vi "Record location.vi"() -> ()   [LabVIEW 2016]
uses:
  Classes/Controllers/Camera/Copy of Camera Folder/Machine Vision.ctl
  Classes/Controllers/Motion/Copy of A3200 Folder/A3200.lvclass
  <vilib>/Utility/file.llb/Read Delimited Spreadsheet (DBL).vi
  <vilib>/Utility/file.llb/Write Delimited Spreadsheet (DBL).vi
  Classes/Controllers/Motion/Copy of Motion Folder/Motion.lvclass
  Classes/Controllers/Camera/Copy of Camera Folder/Camera.lvclass
  Classes/Controllers/Camera/Copy of Controller Folder/Controller.lvclass
panel:
  out "Sum 2":dbl[](array[numeric])
  out "Gantry 2":dbl[](array[numeric])
  out "Camera 2":dbl[](array[numeric])
  in  "Record":bool
  out "XYZTheta Out":dbl[](array[numeric])
  in  "stop":bool
  in  "start":bool
  in  "Speed 1":dbl
  out "XYZTheta Out 2":dbl[](array[numeric])
  in  "file path":path
  out "first row":dbl[](array[numeric])
  out "all rows":dbl[][](array[numeric])
  in  "Z Go":bool
  in  "Position":dbl
  in  "Go":bool
  in  "XYZTheta":dbl[](array[numeric])
  in  "Joystick":bool
  out "Gantry":dbl[](array[numeric])
  out "Sum":dbl[](array[numeric])
  in  "Stop":bool
  out "Image":T1(plugin-control)
  out "Camera":dbl[](array[numeric])
  in  "Machine Vision":T2=enum."None"
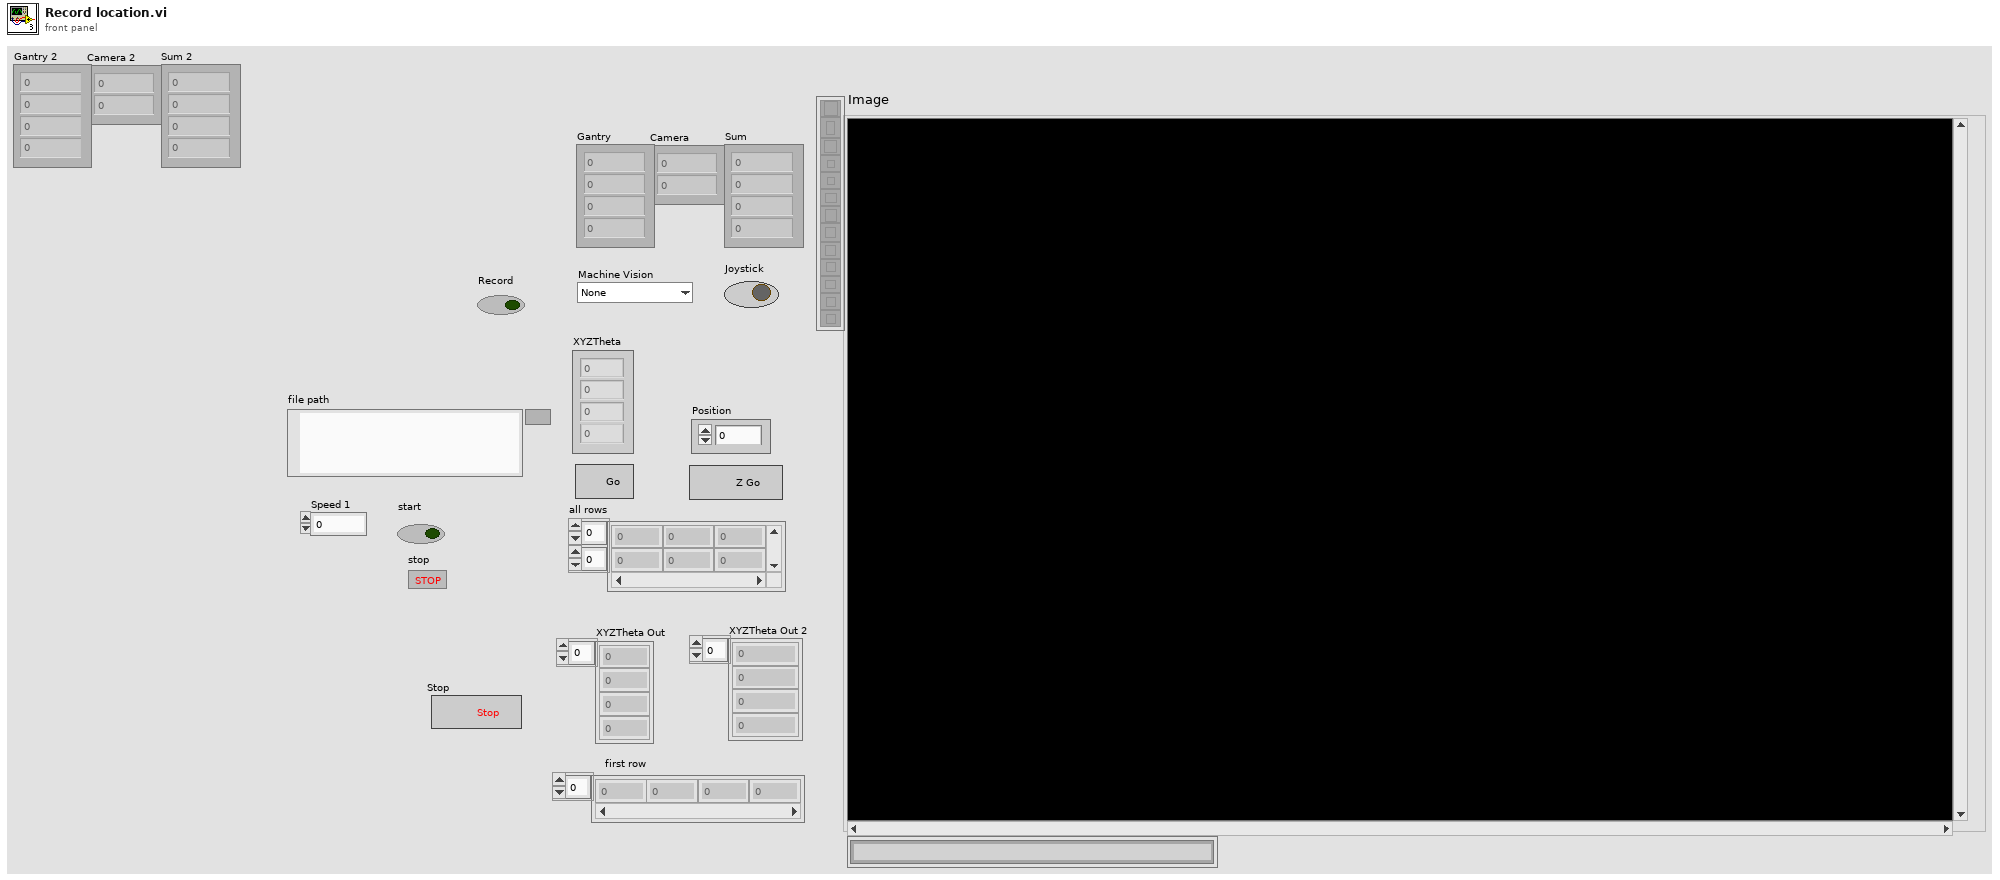
[diagram p1: front panel]
types:
  T1 = typedef "IMAQ Image.ctl" = refnum<image>
  T2 = typedef "Camera.lvclass/Machine Vision.ctl" = enum16{"Focus", "LargeCircle", "None", "INTT HDI Mark", "INTT Sensor Cross", "INTT Chip Corner", "HPK Silicon", "circle"}
  T3 = typedef "Controller.lvclass/Controllers.ctl" = cluster{"Copy of Motion.lvclass":refnum<class "Motion.lvclass">, "Copy of I-O.lvclass":refnum<class "I-O.lvclass">, "Copy of Dispenser.lvclass":refnum<class "Dispenser.lvclass">}
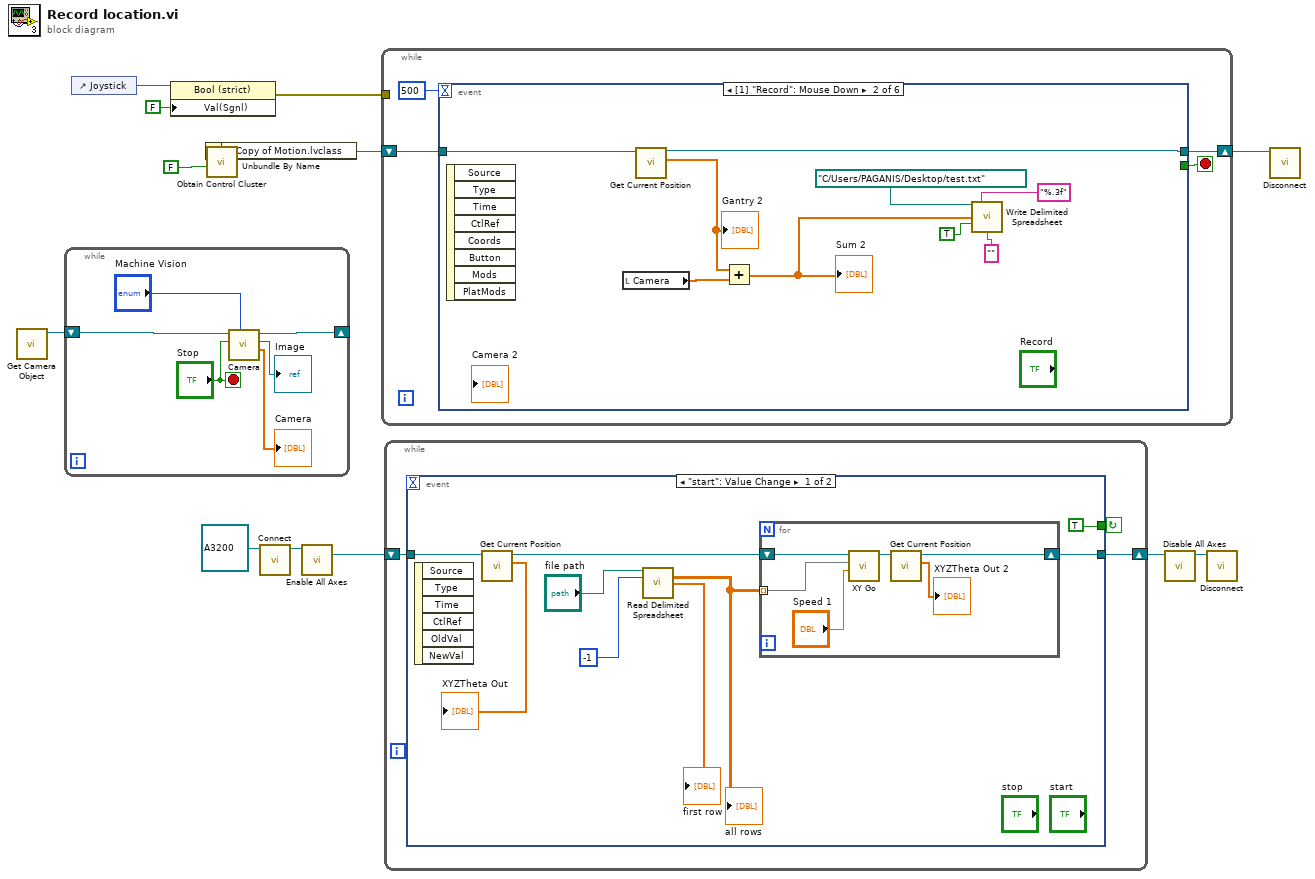
[diagram p0: block diagram]
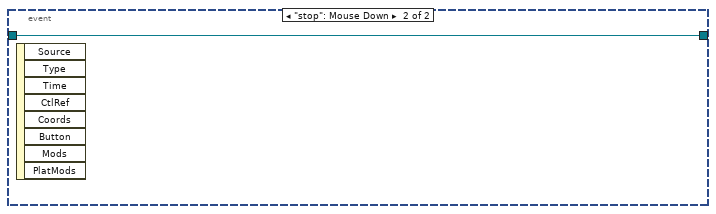
[diagram p2: hidden frame]
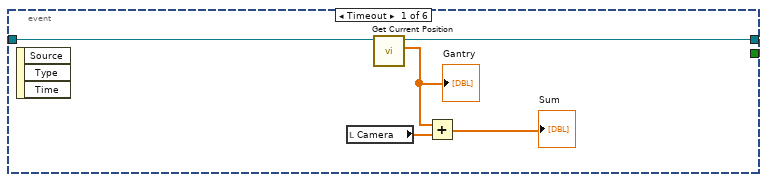
[diagram p3: hidden frame]
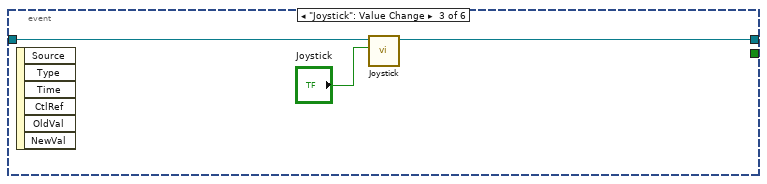
[diagram p4: hidden frame]
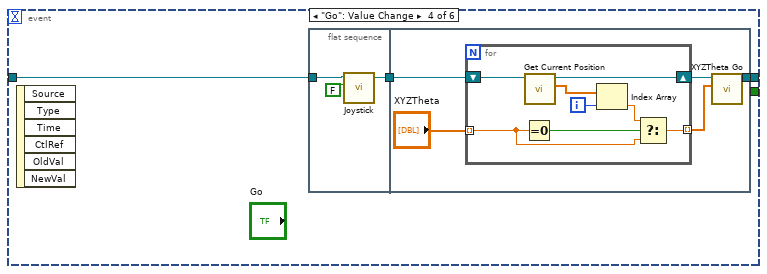
[diagram p5: hidden frame]
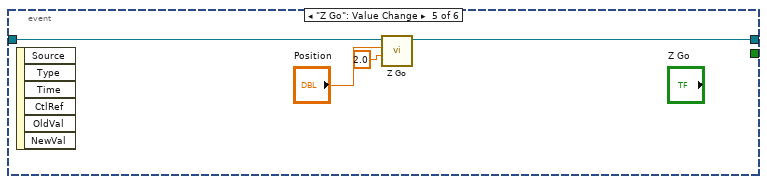
[diagram p6: hidden frame]
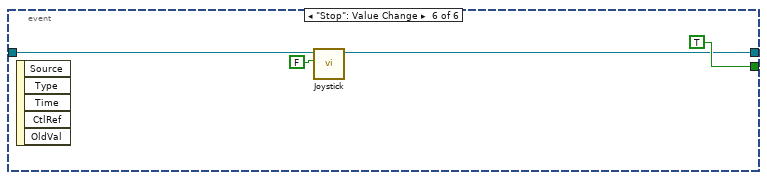
[diagram p7: hidden frame]
diagram:
  n1 = call "Get Camera Object.vi"() -> ("Camera out"=w6:refnum<class "Camera.lvclass">)  [unwired: 10 in, 1 out]
  n2 = while {
    shift-right: [w18] -> _
    shift-left: w6 -> [w19]
    stop <- "Stop" stop-if-true
    n3 = call "Camera.vi"("Machine Vision"="Machine Vision", "Stop"="Stop", "Camera in"=w19) -> ("Camera"=→"Camera":dbl[], "Image"=→"Image":T1, "Camera out"=w18:refnum<class "Camera.lvclass">)  [unwired: 3 in, 3 out]
  }
  n4 = control-ref of="Joystick"() -> (w12:refnum<vi>)
  n5 = property class="Bool (strict)"(reference=w12, "Val(Sgnl)"=FALSE ("Value (Signaling)")) -> (error out=w10:errorcluster)  [unwired: 1 in, 1 out]
  n6 = call "Obtain Control Cluster.vi"("I/O"=FALSE) -> ("Control Out"=w8:T3)  [unwired: 10 in]
  n7 = Unbundle By Name(w8) -> ("Copy of Motion.lvclass"=w7:refnum<class "Motion.lvclass">)
  n8 = call-dynamic "Connect.vi"("Gantry in"=refnum<class "A3200.lvclass"> refnum ("Copy of A3200.lvclass")) -> ("Gantry out"=w4:refnum<class "A3200.lvclass">)  [unwired: 9 in, 1 out]
  n9 = call-dynamic "Enable All Axes.vi"("A3200 in"=w4) -> ("A3200 out"=w3:refnum<class "A3200.lvclass">)  [unwired: 9 in, 1 out]
  n10 = while {
    shift-right: [w20] -> w11
    shift-left: w7 -> [w21]
    tunnel: w10 -> [_]
    stop <- w22 stop-if-true
    n11 = event shown="[1] \"Record\": Mouse Down" {
      selector: _ -> [_ _ _ _ _ _]
      dyn-events: _ -> [_ _ _ _ _ _]
      timeout: 500 -> [_ _ _ _ _ _]
      tunnel: [_ _ _ _ _ TRUE] -> w22
      tunnel: w21 -> [w27 w32 w40 w43 w63 w66]
      tunnel: [w25 w31 w38 w42 w62 w64] -> w20
      event Timeout {
        n12 = event-data() -> ()  [unwired: 1 in, 3 out]
        n13 = local read "Camera"() -> (w28:dbl[])
        n14 = call-dynamic "Get Current Position.vi"("Motion in"=w27) -> ("XYZTheta Out"=w26:dbl[], "Motion out"=w25:refnum<class "Motion.lvclass">)  [unwired: 8 in, 1 out]
        "Gantry" <- w26
        n15 = Add(x=w26, y=w28) -> (x+y=→"Sum":dbl[])
      }
      event "Record": Mouse Down {
        n16 = event-data() -> ()  [unwired: 1 in, 8 out]
        n17 = local read "Camera"() -> (w37:dbl[])
        n18 = call-dynamic "Get Current Position.vi"("Motion in"=w32) -> ("XYZTheta Out"=w36:dbl[], "Motion out"=w31:refnum<class "Motion.lvclass">)  [unwired: 8 in, 1 out]
        "Gantry 2" <- w36
        n19 = Add(x=w36, y=w37) -> (x+y=w29:dbl[])
        "Sum 2" <- w29
        n20 = call-poly <vilib>:"Write Delimited Spreadsheet.vi"("file path (dialog if empty)"=path "C:/Users/PAGANIS/Desktop/test.txt", "format (%.3f)"="%.3f", "1D data"=w29, "append to file? (new file:F)"=TRUE, "delimiter (\\t)"="" ("delimiter (\\t)")) -> ()  [unwired: 9 in, 2 out]
      }
      event "Joystick": Value Change {
        n21 = event-data() -> ()  [unwired: 1 in, 6 out]
        n22 = call-dynamic "Joystick.vi"("Joystick"="Joystick", "Motion in"=w40) -> ("Motion out"=w38:refnum<class "Motion.lvclass">)  [unwired: 8 in, 1 out]
      }
      event "Go": Value Change {
        n23 = event-data() -> ()  [unwired: 1 in, 6 out]
        n24 = flat-sequence {
          tunnel: w43 -> [w45]
          tunnel: [w44] -> w41
          tunnel: [w47] -> w42
          tunnel: w41 -> [w50]
          frame #0 {
            n25 = call-dynamic "Joystick.vi"("Joystick"=FALSE, "Motion in"=w45) -> ("Motion out"=w44:refnum<class "Motion.lvclass">)  [unwired: 8 in, 1 out]
          }
          frame #1 {
            n26 = for {
              tunnel: "XYZTheta" -> [w57] mode=indexing
              tunnel: [w55] -> w49 mode=indexing
              shift-right: [w53] -> w48
              shift-left: w50 -> [w54]
              i -> [w59]
              n27 = Equal To 0?(x=w57) -> (x = 0?=w58:bool)
              n28 = call-dynamic "Get Current Position.vi"("Motion in"=w54) -> ("XYZTheta Out"=w52:dbl[], "Motion out"=w53:refnum<class "Motion.lvclass">)  [unwired: 8 in, 1 out]
              n29 = Index Array(array=w52, index=w59) -> (element=w56:dbl)
              n30 = Select(t=w56, s=w58, f=w57) -> (s? t:f=w55:dbl)
            }
            n31 = call "XYZTheta Go.vi"("XYZTheta In"=w49, "Motion in"=w48) -> ("Motion out"=w47:refnum<class "Motion.lvclass">)  [unwired: 7 in, 2 out]
          }
        }
      }
      event "Z Go": Value Change {
        n32 = event-data() -> ()  [unwired: 1 in, 6 out]
        n33 = call-dynamic "Z Go.vi"("Speed"=2.0, "Position"="Position", "Motion in"=w63) -> ("Motion out"=w62:refnum<class "Motion.lvclass">)  [unwired: 7 in, 1 out]
      }
      event "Stop": Value Change {
        n34 = event-data() -> ()  [unwired: 1 in, 5 out]
        n35 = call-dynamic "Joystick.vi"("Joystick"=FALSE, "Motion in"=w66) -> ("Motion out"=w64:refnum<class "Motion.lvclass">)  [unwired: 8 in, 1 out]
      }
    }
  }
  n36 = while {
    shift-right: [w70] -> w2
    shift-left: w3 -> [w69]
    stop <- w68 continue-if-true
    n37 = event shown="[0] \"start\": Value Change" {
      selector: _ -> [_ _]
      dyn-events: _ -> [_ _]
      timeout: _ -> [_ _]
      tunnel: [w79 w86] -> w70
      tunnel: w69 -> [w77 w86]
      tunnel: [TRUE _] -> w68
      event "start": Value Change {
        n38 = event-data() -> ()  [unwired: 1 in, 6 out]
        n39 = call-dynamic "Get Current Position.vi"("Gantry in"=w77) -> ("XYZTheta Out"=→"XYZTheta Out":dbl[], "Gantry out"=w76:refnum<class "A3200.lvclass">)  [unwired: 8 in, 1 out]
        n40 = call-poly <vilib>:"Read Delimited Spreadsheet.vi"("file path (dialog if empty)"="file path", "number of rows (all:-1)"=-1) -> ("all rows"=w71:dbl[][], "first row"=→"first row":dbl[])  [unwired: 8 in, 4 out]
        "all rows" <- w71
        n41 = for {
          shift-right: [w83] -> w79
          shift-left: w76 -> [w81]
          tunnel: w71 -> [w80] mode=indexing
          n42 = call-dynamic "XY Go.vi"("Speed"="Speed 1", "XY"=w80, "Gantry in"=w81) -> ("Gantry out"=w84:refnum<class "A3200.lvclass">)  [unwired: 7 in, 1 out]
          n43 = call-dynamic "Get Current Position.vi"("Gantry in"=w84) -> ("XYZTheta Out"=→"XYZTheta Out 2":dbl[], "Gantry out"=w83:refnum<class "A3200.lvclass">)  [unwired: 8 in, 1 out]
        }
      }
      event "stop": Mouse Down {
        n44 = event-data() -> ()  [unwired: 1 in, 8 out]
      }
    }
  }
  n45 = call-dynamic "Disable All Axes.vi"("Gantry in"=w2) -> ("Gantry out"=w1:refnum<class "A3200.lvclass">)  [unwired: 9 in, 1 out]
  n46 = call-dynamic "Disconnect.vi"("Gantry in"=w1) -> ()  [unwired: 9 in, 1 out]
  n47 = call-dynamic "Disconnect.vi"("Controller in"=w11) -> ()  [unwired: 9 in, 1 out]
